vi "Voltage vs time.vi"() -> ()   [LabVIEW 2021]
panel:
  in  "minimum value":dbl=-5.0 format="%0.2f"
  in  "maximum value":dbl=5.0 format="%0.2f"
  in  "physical channels":tag="Dev1/ai1"
  in  "Combo Box":string(combo)="NIDAQ"
  in  "Stop":bool
  out "XY Graph":cluster{dbl[], dbl[]}(graph)
  in  "Delay Time (s)":dbl=300.0
  in  "MDO 3034 VISA":refnum<visa-resource-name>="USB0::0x0699::0x0408::C047957::INSTR"
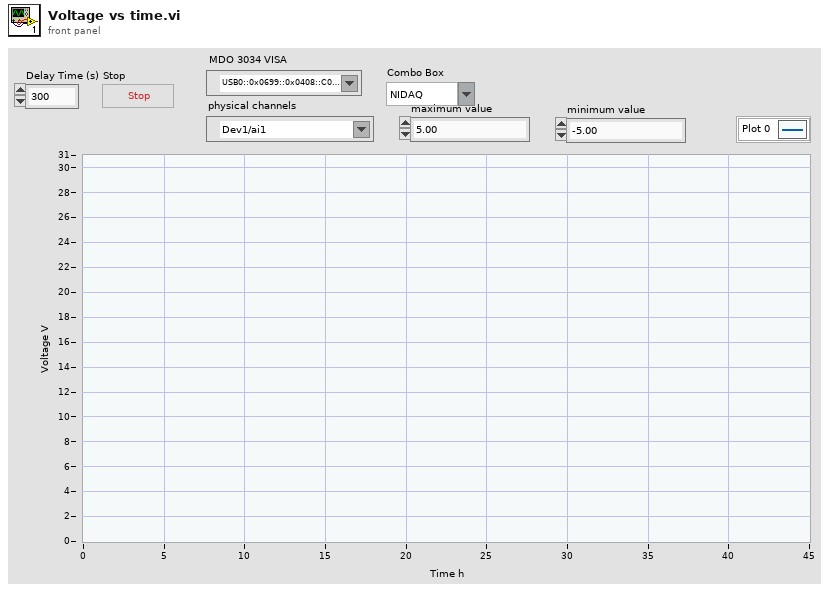
[diagram p1: front panel]
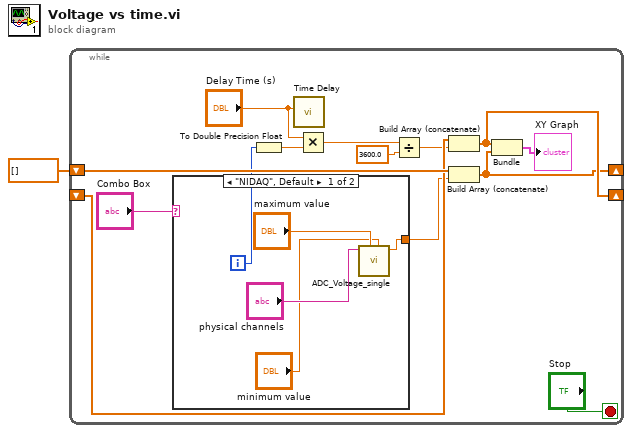
[diagram p0: block diagram]
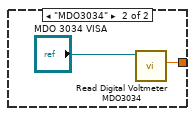
[diagram p2: hidden frame]
diagram:
  n1 = while {
    shift-right: [w9] -> _
    shift-left: dbl[] [] -> [w15]
    shift-right: [w10] -> _
    shift-left: _ -> [w11]
    i -> [w14]
    stop <- "Stop" stop-if-true
    n2 = case shown="\"NIDAQ\", Default" "Combo Box" {
      tunnel: [w18 w21] -> w6
      frame "NIDAQ", Default {
        n3 = call "ADC_Voltage_single.vi"("minimum value"="minimum value", "maximum value"="maximum value", "physical channels"="physical channels") -> ("data"=w18:dbl)  [unwired: 7 in, 1 out]
      }
      frame "MDO3034" {
        n4 = call "Read Digital Voltmeter MDO3034.vi"("VISA resource name"="MDO 3034 VISA") -> ("Digital Voltmeter Value"=w21:dbl)  [unwired: 8 in, 2 out]
      }
    }
    n5 = To Double Precision Float(number=w14) -> (double precision float=w12:dbl)
    n6 = call "Time Delay"("Delay Time (s)"="Delay Time (s)") -> ()  [unwired: 10 in, 1 out]
    n7 = Multiply(x="Delay Time (s)", y=w12) -> (x*y=w4:dbl)
    n8 = Divide(x=w4, y=3600.0) -> (x/y=w5:dbl)
    n9 = Build Array (concatenate)(w11, w5) -> (w10:dbl[])
    n10 = Build Array (concatenate)(w15, w6) -> (w9:dbl[])
    n11 = Bundle(w10, w9) -> (→"XY Graph":cluster{dbl[], dbl[]})  [unwired: 1 in]
  }
